vi "state machine.vi"() -> ()   [LabVIEW 2018, in "state machine.lvlib"]
uses:
  state machine.lvlib
  <vilib>/eio/EIONode/EIONode.xnode
  <vilib>/rvi/eio/common/nirviEmuTemplateMethod_errors.vi
  states.ctl
  <vilib>/Platform/TimedLoop/XDataNode/XDataNode.xnode
  <vilib>/Platform/TimedLoop/XDataNode/nitl_modes.ctl
  <vilib>/Platform/TimedLoop/XDataNode/XDNodeRunTimeDep.lvlib
  <vilib>/Platform/TimedLoop/XDataNode/wakeup.ctl
  <vilib>/Platform/TimedLoop/XDataNode/timing_clust.ctl
  shutter-modes.ctl
  scan param.ctl
panel:
  in  "scan param":T1
  out "curr state":T3
  out "counts":u32[](array[numeric])
  out "APDs pre-pixel":u32[](array[numeric])
  out "APDs":u32[](array[numeric])
  in  "stop":bool
  out "pixel counter":i16
  in  "line go!":bool
  in  "states":T3
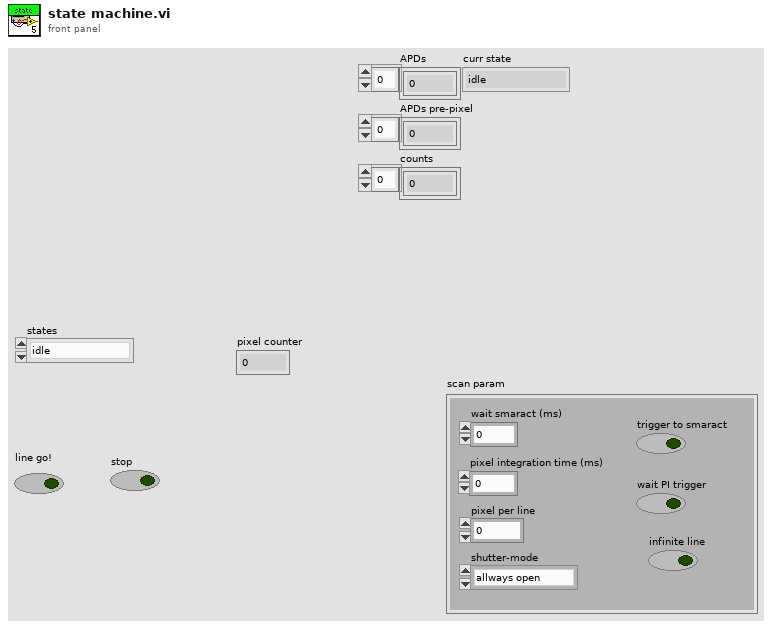
[diagram p1: front panel]
types:
  T1 = typedef "state machine.lvlib/scan param.ctl" = cluster{"wait smaract (us)":u32, "pixel integration time (us)":u32, "pixel per line":i16, "shutter-mode":T2, "trigger to smaract":bool, "wait PI trigger":bool, "infinite line":bool}
  T2 = typedef "state machine.lvlib/shutter-modes.ctl" = enum16{"allways open", "allways closed", "open per line", "open per pixel"}
  T3 = typedef "state machine.lvlib/states.ctl" = enum16{"idle", "pre-line", "pre-pixel", "pixel-integration", "pixel-readout", "post-pixel", "post-line"}
  T4 = typedef "XDNodeRunTimeDep.lvlib/timing_clust.ctl" = cluster{"Expected End [f-1]":u64, "Actual End [f-1]":u64, "Finished Late? [f-1]":bool, "Expected End [i-1]":u64, "Actual End [i-1]":u64, "Finished Late? [i-1]":bool, "Expected Start [i]":u64, "Actual Start [i]":u64, "Expected Start [f]":u64, "Actual Start [f]":u64, "Source Name":string, "Structure Name":string, "Period":i64, "Deadline":i64, "Offset":i64, "Start":i64, "Priority":i32, "Timeout":i32, "Mode":T5, "Wakeup Reason":T6, "Error":errorcluster, "Source Type":string, "Secondary Source Type":string, "Global End Time":u64, "Global Start Time":u64, "Frame Duration":u64, "Iteration Duration":u64, "Assigned CPU":i32, "I/O Scan Engine Mode":u32}
  T5 = typedef "XDNodeRunTimeDep.lvlib/nitl_modes.ctl" = enum32{"No Change", "Process missed periods, maintain original phase", "Discard missed periods, maintain original phase", "Process missed periods, ignore original phase", "Discard missed periods, ignore original phase"}
  T6 = typedef "XDNodeRunTimeDep.lvlib/wakeup.ctl" = enum32{"Normal", "Aborted", "Asynchronous wakeup", "Timing source error", "Timed loop error", "Timeout"}
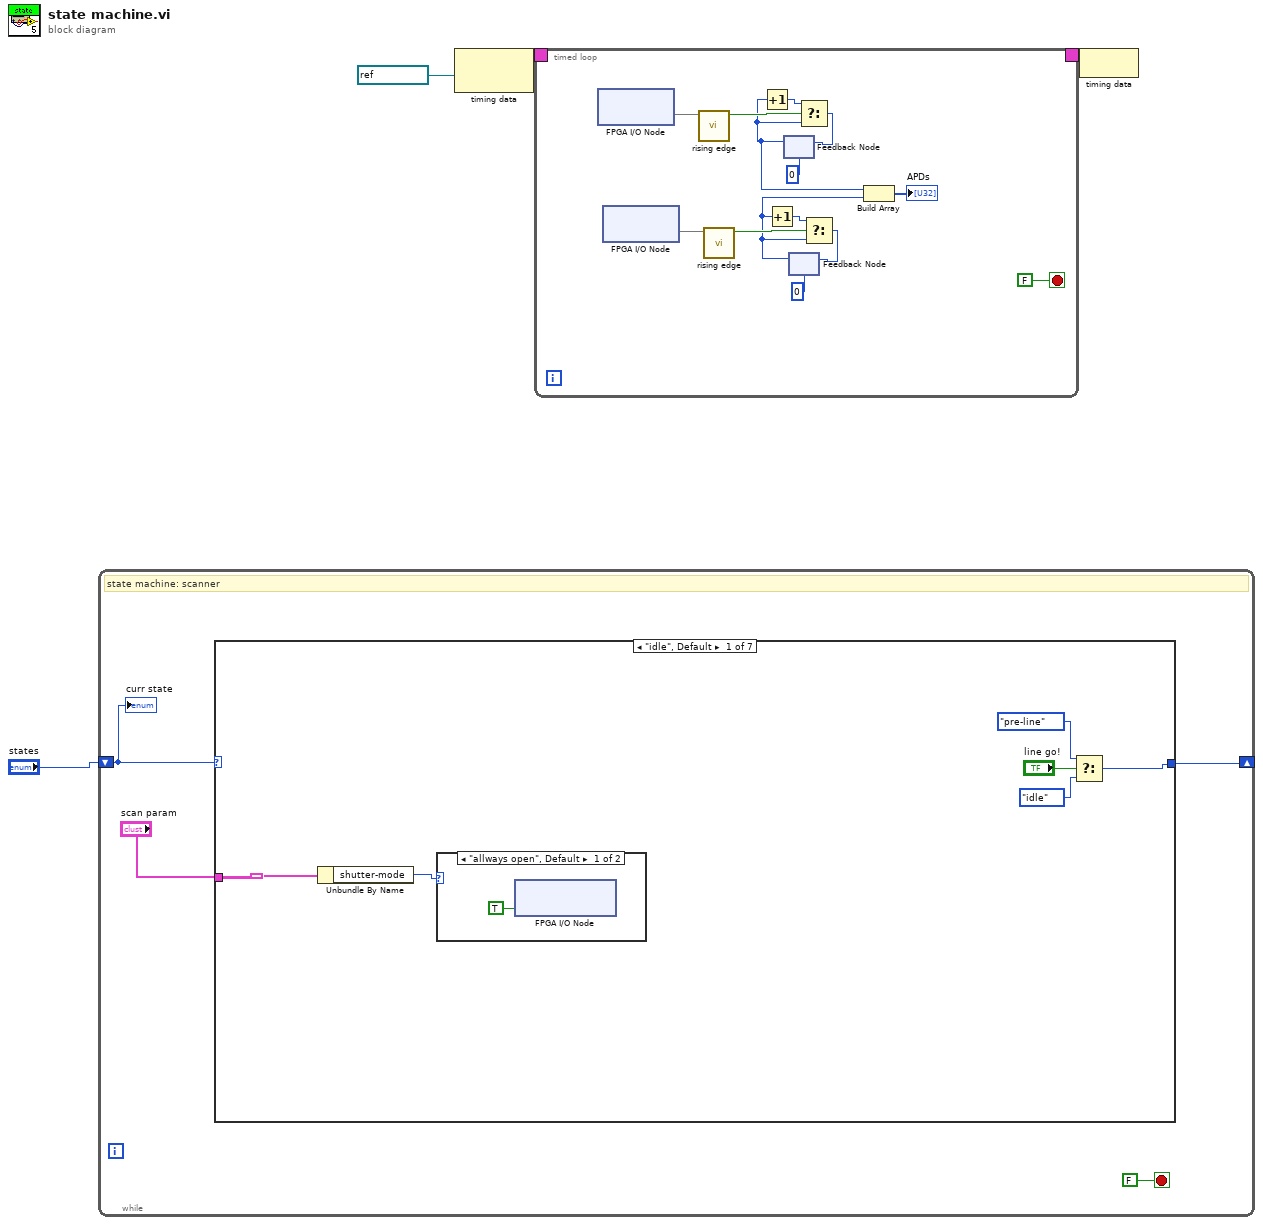
[diagram p0: block diagram]
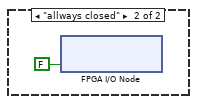
[diagram p2: hidden frame]
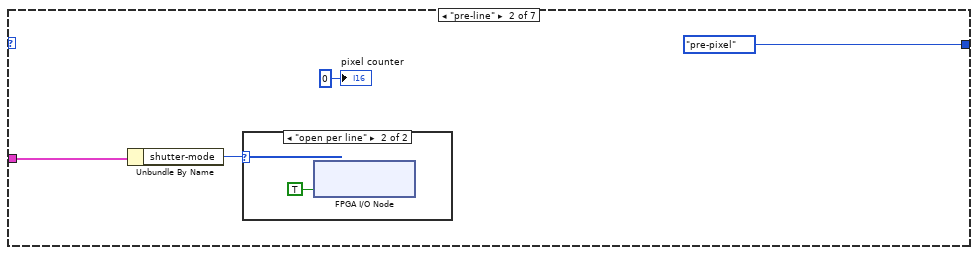
[diagram p3: hidden frame]
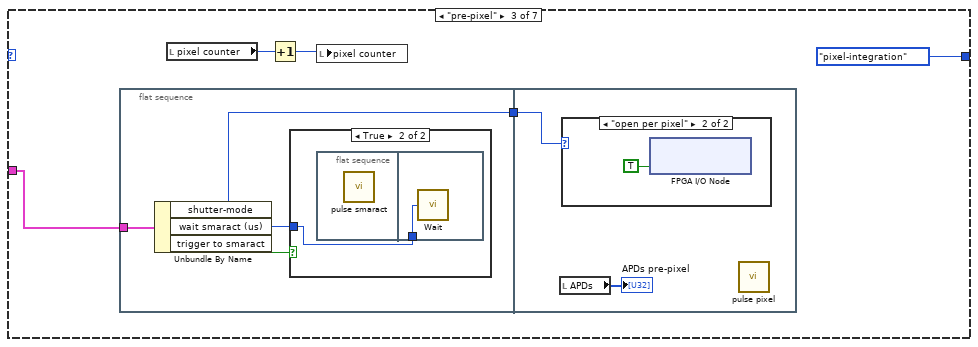
[diagram p5: hidden frame]
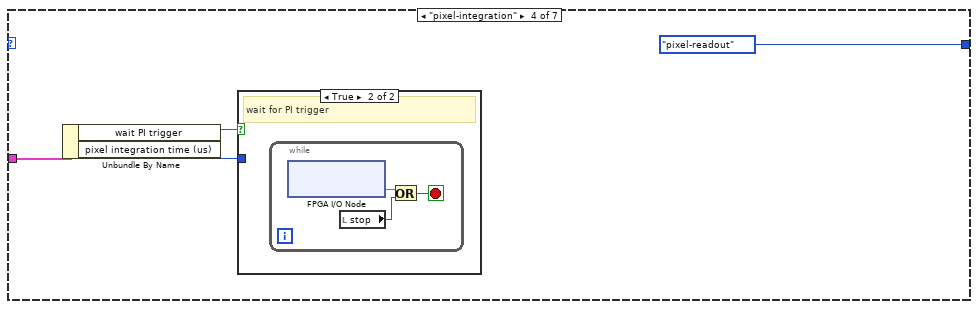
[diagram p8: hidden frame]
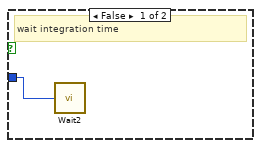
[diagram p9: hidden frame]
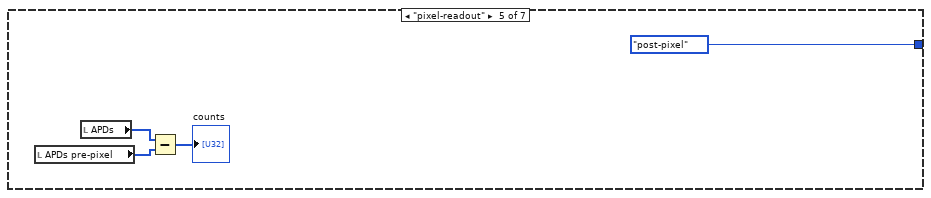
[diagram p10: hidden frame]
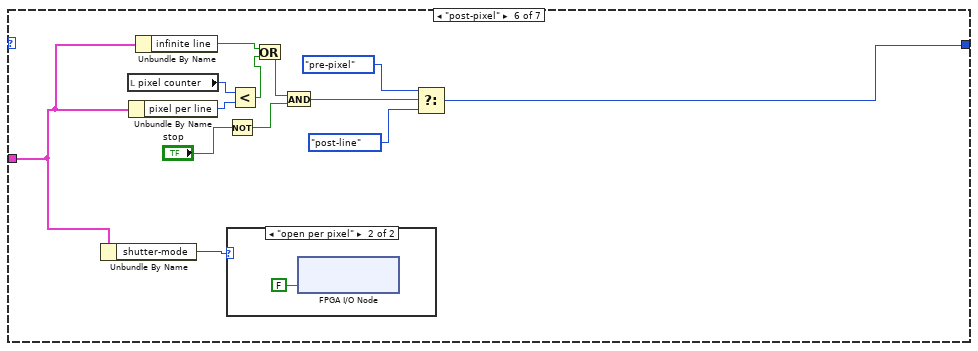
[diagram p11: hidden frame]
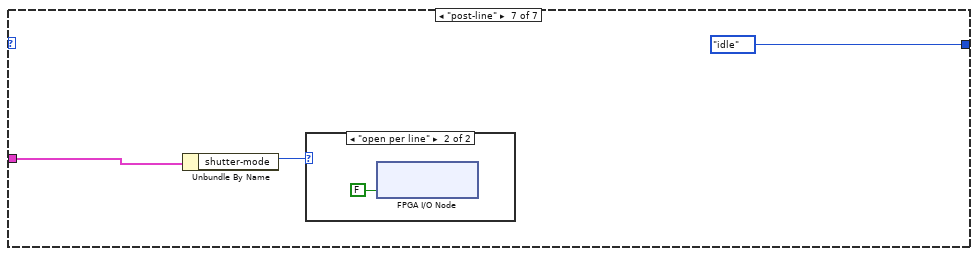
[diagram p13: hidden frame]
diagram:
  n1 = while {
    shift-right: [w7] -> _
    shift-left: "states" -> [w6]
    stop <- FALSE stop-if-true
    # "state machine: scanner"
    n2 = case shown="\"idle\", Default" w6 {
      tunnel: [w13 states."pre-pixel" ("states") states."pixel-integration" ("states") states."pixel-readout" ("states") states."post-pixel" ("states") w56 states."idle" ("states")] -> w7
      tunnel: "scan param" -> [w9 w17 w23 w38 _ w51 w62]
      frame "idle", Default {
        n3 = Unbundle By Name(w9) -> ("shutter-mode"=w10:T2)
        n4 = case shown="\"allways open\", Default" w10 {
          frame "allways open", Default {
            n5 = xnode "FPGA I/O Node"("shutter out"=TRUE) -> ()  [unwired: 1 in, 1 out]
          }
          frame "allways closed" {
            n6 = xnode "FPGA I/O Node"("shutter out"=FALSE) -> ()  [unwired: 1 in, 1 out]
          }
        }
        n7 = Select(t=states."pre-line" ("states"), s="line go!", f=states."idle" ("states")) -> (s? t:f=w13:T3)
      }
      frame "pre-line" {
        n8 = Unbundle By Name(w17) -> ("shutter-mode"=w18:T2)
        n9 = case shown="\"open per line\"" w18 {
          frame "allways open", Default {
          }
          frame "open per line" {
            n10 = xnode "FPGA I/O Node"("shutter out"=TRUE) -> ()  [unwired: 1 in, 1 out]
          }
        }
        "pixel counter" <- i16 0 ("pixel counter")
      }
      frame "pre-pixel" {
        n11 = flat-sequence {
          tunnel: [w30] -> w22
          tunnel: w23 -> [w29]
          tunnel: w22 -> [w33]
          frame #0 {
            n12 = Unbundle By Name(w29) -> ("shutter-mode"=w30:T2, "wait smaract (us)"=w27:u32, "trigger to smaract"=w28:bool)
            n13 = case shown="True" w28 {
              tunnel: w27 -> [_ w31]
              frame False {
              }
              frame True {
                n14 = flat-sequence {
                  tunnel: w31 -> [w32]
                  frame #0 {
                    n15 = call "pulse smaract.vi"() -> ()  [unwired: 12 in]
                  }
                  frame #1 {
                    n16 = call "Wait"("Count(mSec)"=w32) -> ()  [unwired: 1 out]
                  }
                }
              }
            }
          }
          frame #1 {
            n17 = local read "APDs"() -> (→"APDs pre-pixel":u32[])
            n18 = case shown="\"open per pixel\"" w33 {
              frame "allways open", Default {
              }
              frame "open per pixel" {
                n19 = xnode "FPGA I/O Node"("shutter out"=TRUE) -> ()  [unwired: 1 in, 1 out]
              }
            }
            n20 = call "pulse pixel.vi"() -> ()  [unwired: 12 in]
          }
        }
        n21 = local read "pixel counter"() -> (w26:i16)
        n22 = Increment(x=w26) -> (x+1=w25:i16)
        n23 = local write "pixel counter"(w25) -> ()
      }
      frame "pixel-integration" {
        n24 = Unbundle By Name(w38) -> ("wait PI trigger"=w37:bool, "pixel integration time (us)"=w36:u32)
        n25 = case shown="True" w37 {
          tunnel: w36 -> [w40 _]
          frame False {
            # "wait integration time"
            n26 = call "Wait2"("Count(mSec)"=w40) -> ()  [unwired: 1 out]
          }
          frame True {
            # "wait for PI trigger"
            n27 = while {
              stop <- w43 stop-if-true
              n28 = xnode "FPGA I/O Node"() -> ("PI stage in"=w42)  [unwired: 1 in, 1 out]
              n29 = local read "stop"() -> (w41:bool)
              n30 = Or(x=w42, y=w41) -> (x .or. y?=w43:bool)
            }
          }
        }
      }
      frame "pixel-readout" {
        n31 = local read "APDs pre-pixel"() -> (w45:u32[])
        n32 = local read "APDs"() -> (w46:u32[])
        n33 = Subtract(x=w46, y=w45) -> (x-y=→"counts":u32[])
      }
      frame "post-pixel" {
        n34 = Unbundle By Name(w51) -> ("shutter-mode"=w53:T2)
        n35 = local read "pixel counter"() -> (w60:i16)
        n36 = Unbundle By Name(w51) -> ("pixel per line"=w52:i16)
        n37 = Unbundle By Name(w51) -> ("infinite line"=w50:bool)
        n38 = Not(x="stop") -> (.not. x?=w58:bool)
        n39 = case shown="\"open per pixel\"" w53 {
          frame "allways open", Default {
          }
          frame "open per pixel" {
            n40 = xnode "FPGA I/O Node"("shutter out"=FALSE) -> ()  [unwired: 1 in, 1 out]
          }
        }
        n41 = Less?(x=w60, y=w52) -> (x < y?=w49:bool)
        n42 = Or(x=w50, y=w49) -> (x .or. y?=w48:bool)
        n43 = And(x=w48, y=w58) -> (x .and. y?=w57:bool)
        n44 = Select(t=states."pre-pixel" ("states"), s=w57, f=states."post-line" ("states")) -> (s? t:f=w56:T3)
      }
      frame "post-line" {
        n45 = Unbundle By Name(w62) -> ("shutter-mode"=w63:T2)
        n46 = case shown="\"open per line\"" w63 {
          frame "allways open", Default {
          }
          frame "open per line" {
            n47 = xnode "FPGA I/O Node"("shutter out"=FALSE) -> ()  [unwired: 1 in, 1 out]
          }
        }
      }
    }
    "curr state" <- w6
  }
  n48 = node-c288(refnum<k21> "240MHz" ("Source Name")) -> (w3:T4)
  n49 = timed-loop {
    timing: w3 -> [_]
    timing-out: [_] -> w2
    stop <- FALSE stop-if-true
    n50 = xnode "FPGA I/O Node"() -> ("APD1"=w78)  [unwired: 1 in, 1 out]
    n51 = xnode "FPGA I/O Node"() -> ("APD2"=w74)  [unwired: 1 in, 1 out]
    n52 = call "rising edge.vi"("APD1"=w78) -> ("Boolean"=w77:bool)  [unwired: 10 in]
    n53 = call "rising edge.vi"("APD1"=w74) -> ("Boolean"=w73:bool)  [unwired: 10 in]
    n54 = feedback #1(u32 0) -> (w68:u32)
    n55 = Increment(x=w68) -> (x+1=w76:u32)
    n56 = feedback #2(u32 0) -> (w67:u32)
    n57 = Increment(x=w67) -> (x+1=w72:u32)
    n58 = Select(t=w76, s=w77, f=w68) -> (s? t:f=w69:u32)
    n59 = feedback-in #1(w69) -> ()
    n60 = Select(t=w72, s=w73, f=w67) -> (s? t:f=w70:u32)
    n61 = feedback-in #2(w70) -> ()
    n62 = Build Array(w68, w67) -> (→"APDs":u32[])
  }
  n63 = node-c288(w2) -> ()
